vi "Main.vi"() -> ()   [LabVIEW 2014]
uses:
  SubVIs/States.ctl
panel:
  out "Table":string[][](table)
  out "Player Name":string caption="Name"
  out "Signal Wave":waveform(dbl)(graph) caption="Sine with Uniform Noise"
  out "Attempts":u32
  in  "Resest Button":bool
  in  "stop":bool
  in  "Play Button":bool
  out "Glass Status":dbl(slide) scale=0.0..10.0
  in  "Hit Button":bool
  in  "Power":dbl(slide) scale=0.0..10.0
  # "Broken!"
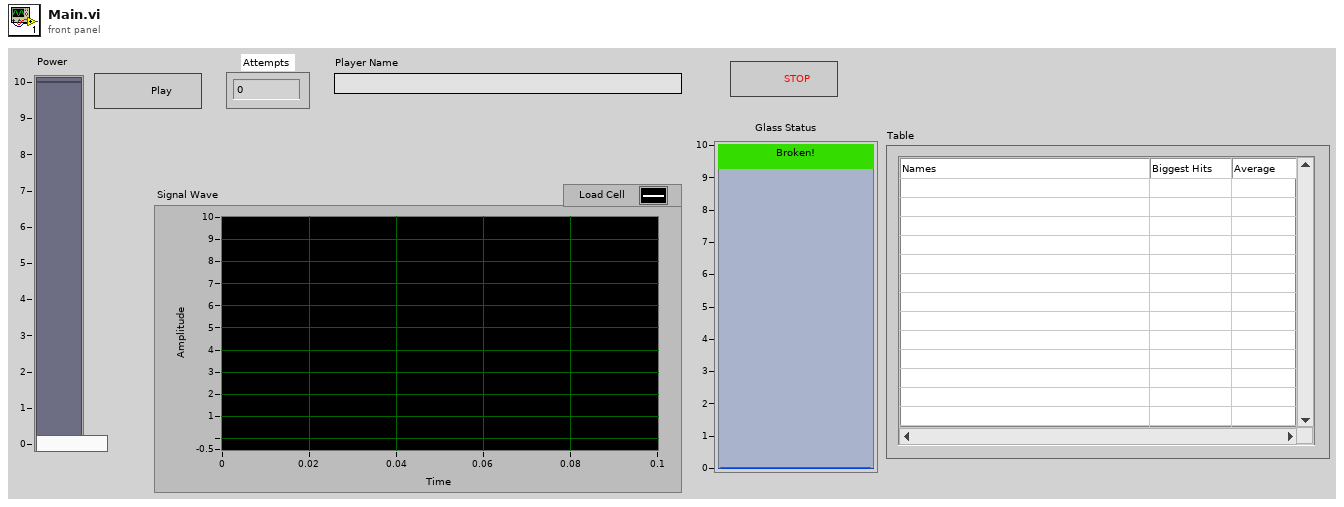
[diagram p1: front panel]
types:
  T1 = typedef "States.ctl" = enum16{"Wait to Start", "Run", "Hit", "Check Glass Status", "Glass Broken", "Stats", "Game Over"}
  T2 = cluster{"Name":string, "Biggest Hit":dbl, "Average":dbl}
  T3 = enum16{"Left Button", "Center Button", "Right Button", "Window Close"}
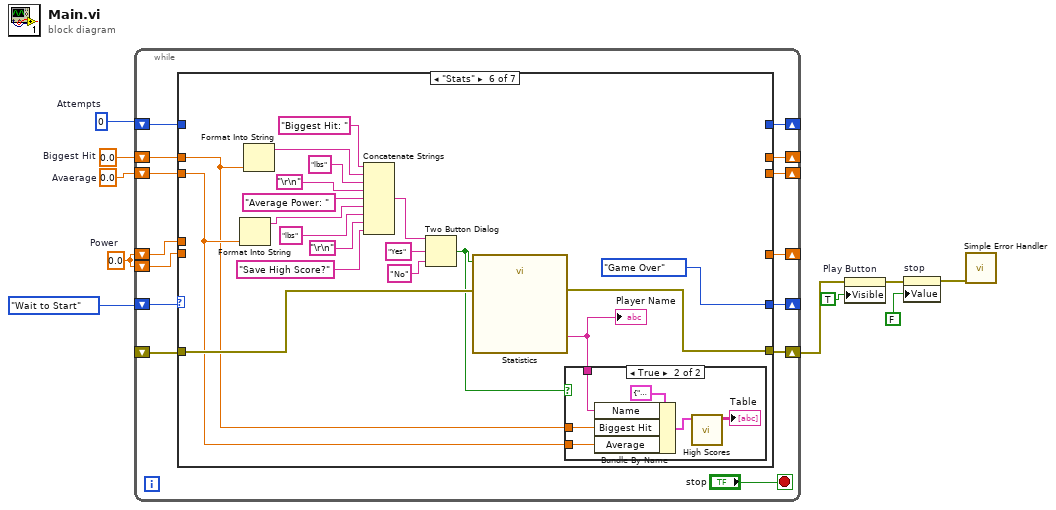
[diagram p0: block diagram]
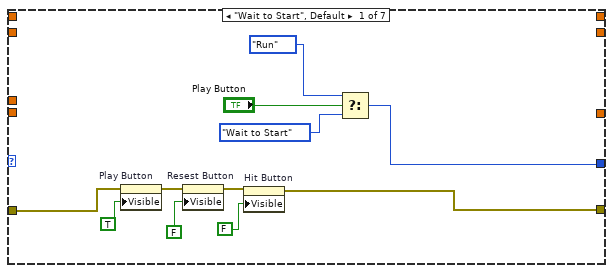
[diagram p2: hidden frame]
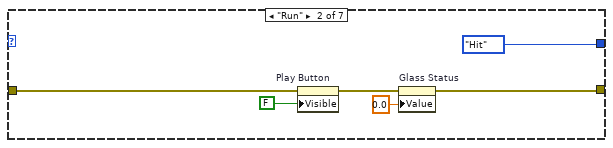
[diagram p3: hidden frame]
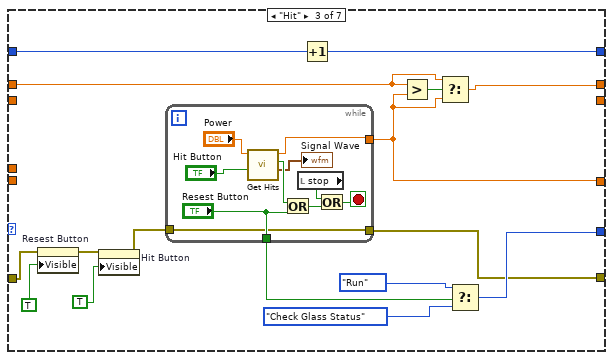
[diagram p4: hidden frame]
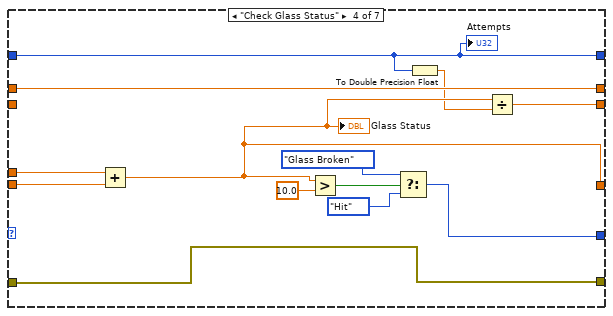
[diagram p5: hidden frame]
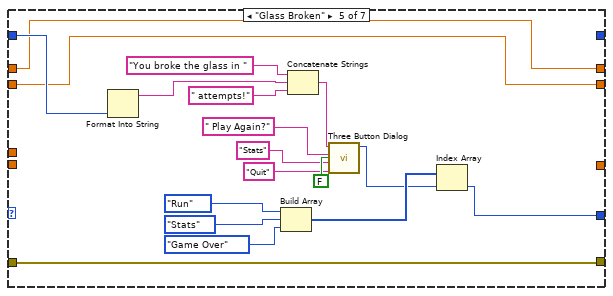
[diagram p6: hidden frame]
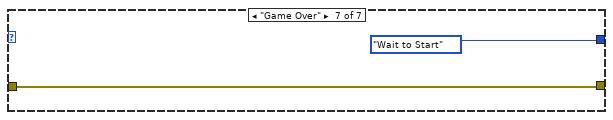
[diagram p8: hidden frame]
diagram:
  w1 = 0.0  # Avaerage
  w2 = 0.0  # Biggest Hit
  w6 = u32 0  # Attempts
  w10 = 0.0  # Power
  n1 = while {
    shift-right: [w24] -> _
    shift-left: w10 -> [w23]
    shift-left: w10 -> [w22]
    shift-right: [w20] -> _
    shift-left: States."Wait to Start" ("States") -> [w21]
    shift-right: [w18] -> w7
    shift-left: _ -> [w17]
    shift-right: [w16] -> _
    shift-left: w6 -> [w15]
    shift-right: [w14] -> _
    shift-left: w2 -> [w13]
    shift-right: [w12] -> _
    shift-left: w1 -> [w11]
    stop <- "stop" stop-if-true
    n2 = case shown="\"Stats\"" w21 {
      tunnel: [_ _ w44 w71 _ _ _] -> w24
      tunnel: w23 -> [_ _ _ w80 _ _ _]
      tunnel: w22 -> [_ _ _ w79 _ _ _]
      tunnel: [w34 States."Hit" ("States") w56 w76 w83 States."Game Over" ("States") States."Wait to Start" ("States")] -> w20
      tunnel: [w28 w38 w51 w75 w98 w116 w125] -> w18
      tunnel: w17 -> [w27 w37 w50 w75 w98 w117 w125]
      tunnel: [_ _ w49 w68 _ _ _] -> w16
      tunnel: w15 -> [_ _ w48 w68 w95 _ _]
      tunnel: [_ _ w42 w72 w82 _ _] -> w14
      tunnel: w13 -> [_ _ w43 w72 w82 w100 _]
      tunnel: [_ _ _ w69 w81 _ _] -> w12
      tunnel: w11 -> [_ _ _ _ w81 w101 _]
      frame "Wait to Start", Default {
        n3 = property on="Play Button" class="Bool"(error in=w27, "Visible"=TRUE) -> (error out=w30:errorcluster)  [unwired: 1 in, 1 out]
        n4 = property on="Resest Button" class="Bool"(error in=w30, "Visible"=FALSE) -> (error out=w32:errorcluster)  [unwired: 1 in, 1 out]
        n5 = property on="Hit Button" class="Bool"(error in=w32, "Visible"=FALSE) -> (error out=w28:errorcluster)  [unwired: 1 in, 1 out]
        n6 = Select(t=States."Run" ("States"), s="Play Button", f=States."Wait to Start" ("States")) -> (s? t:f=w34:T1)
      }
      frame "Run" {
        n7 = property on="Play Button" class="Bool"(error in=w37, "Visible"=FALSE) -> (error out=w40:errorcluster)  [unwired: 1 in, 1 out]
        n8 = property on="Glass Status" class="Slide (strict)"(error in=w40, "Value"=0.0 ("Glass Status")) -> (error out=w38:errorcluster)  [unwired: 1 in, 1 out]
      }
      frame "Hit" {
        n9 = property on="Resest Button" class="Bool"(error in=w50, "Visible"=TRUE) -> (error out=w55:errorcluster)  [unwired: 1 in, 1 out]
        n10 = property on="Hit Button" class="Bool"(error in=w55, "Visible"=TRUE) -> (error out=w52:errorcluster)  [unwired: 1 in, 1 out]
        n11 = while {
          tunnel: [w60] -> w44
          tunnel: ["Resest Button"] -> w57
          tunnel: w52 -> [w63]
          tunnel: [w63] -> w51
          stop <- w65 stop-if-true
          n12 = call "Get Hits.vi"("Hit?"="Hit Button", "Power"="Power") -> ("Load Cell Signal"=→"Signal Wave":waveform(dbl), "Hit? Passed Through"=w59:bool, "Hit Value"=w60:dbl)  [unwired: 7 in]
          n13 = Or(x=w59, y="Resest Button") -> (x .or. y?=w66:bool)
          n14 = local read "stop"() -> (w64:bool)
          n15 = Or(x=w64, y=w66) -> (x .or. y?=w65:bool)
        }
        n16 = Increment(x=w48) -> (x+1=w49:u32)
        n17 = Greater?(x=w43, y=w44) -> (0:w45:bool)
        n18 = Select(t=w43, s=w45, f=w44) -> (s? t:f=w42:dbl)
        n19 = Select(t=States."Run" ("States"), s=w57, f=States."Check Glass Status" ("States")) -> (s? t:f=w56:T1)
      }
      frame "Check Glass Status" {
        n20 = Add(x=w80, y=w79) -> (x+y=w71:dbl)
        "Glass Status" <- w71
        n21 = Greater?(x=w71, y=10.0) -> (0:w78:bool)
        n22 = Select(t=States."Glass Broken" ("States"), s=w78, f=States."Hit" ("States")) -> (s? t:f=w76:T1)
        n23 = To Double Precision Float(number=w68) -> (double precision float=w70:dbl)
        n24 = Divide(x=w71, y=w70) -> (x/y=w69:dbl)
        "Attempts" <- w68
      }
      frame "Glass Broken" {
        n25 = Format Into String(w95) -> (resulting string=w94:string)  [unwired: 3 in, 1 out]
        n26 = Build Array(States."Run" ("States"), States."Stats" ("States"), States."Game Over" ("States")) -> (w85:T1[])
        n27 = Concatenate Strings("You broke the glass in " ("message"), w94, " attempts!" ("string")) -> (w90:string)
        n28 = call <vilib>:"Three Button Dialog.vi"("Allow user to close window? (TRUE)"=FALSE, "Right Button Text (\"Cancel\")"="Quit" ("F button name (\"Cancel\")"), "Center Button Text (\"No\")"="Stats" ("T button name (\"OK\")"), "Left Button Text (\"Yes\")"=" Play Again?" ("string"), "message"=w90) -> ("Which Button?"=w84:T3)  [unwired: 6 in]
        n29 = Index Array(array=w85, index=w84) -> (element=w83:T1)
      }
      frame "Stats" {
        n30 = Format Into String(w101) -> (resulting string=w103:string)  [unwired: 3 in, 1 out]
        n31 = Format Into String(w100) -> (resulting string=w104:string)  [unwired: 3 in, 1 out]
        n32 = Concatenate Strings("Biggest Hit: " ("string"), w104, "lbs" ("string"), "\r\n", "Average Power: " ("string"), w103, "lbs" ("string"), "\r\n", "Save High Score?" ("string")) -> (w110:string)
        n33 = Two Button Dialog(message=w110, 1:"No" ("F button name (\"Cancel\")"), 2:"Yes" ("T button name (\"OK\")")) -> (T button?=w99:bool)
        n34 = call "Statistics"("Enable"=w99, "error in (no error)"=w117) -> ("Name"=w102:string, "error out"=w116:errorcluster)  [unwired: 15 in, 1 out]
        "Player Name" <- w102
        n35 = case shown="True" w99 {
          tunnel: w102 -> [_ w123]
          tunnel: w101 -> [_ w122]
          tunnel: w100 -> [_ w121]
          frame False {
          }
          frame True {
            n36 = Bundle By Name(cluster=T2 {"Name"="", "Biggest Hit"=0.0, "Average"=0.0} ("input cluster"), "Name"=w123, "Biggest Hit"=w121, "Average"=w122) -> (w119:T2)
            n37 = call "High Scores.vi"("Player Data"=w119) -> ("Table"=→"Table":string[][])  [unwired: 10 in]
          }
        }
      }
      frame "Game Over" {
      }
    }
  }
  n38 = property on="Play Button" class="Bool"(error in=w7, "Visible"=TRUE) -> (error out=w5:errorcluster)  [unwired: 1 in, 1 out]
  n39 = property on="stop" class="Bool (strict)"(error in=w5, "Value"=FALSE ("Visible")) -> (error out=w4:errorcluster)  [unwired: 1 in, 1 out]
  n40 = call <vilib>:"Simple Error Handler.vi"("error in (no error)"=w4) -> ()  [unwired: 4 in, 5 out]
